vi "Format Alarm Data.vi"(5 "Area color settings":T3(array[cluster]), 7 "Alarm Display Format":T2(array[ring])=[enum."alarm URL"], 8 "Error In":errorcluster, 10 "alarm instances":T1(array[cluster]), 11 "Multicolumn Listbox":refnum<vi>) -> (0 "Error Out":errorcluster, 1 "Alarm Summary Data":string[][](array[string]), 2 "Alarm Summary Headers":string[](array[string]), 3 "dup Multicolumn Listbox":refnum<vi>)   [LabVIEW 2018, in "Dynamic Shared Variables.lvlib"]
doc: "This VI formats alarm data and inserts it into a multicolumn list box."
uses:
  Dynamic Shared Variables.lvlib
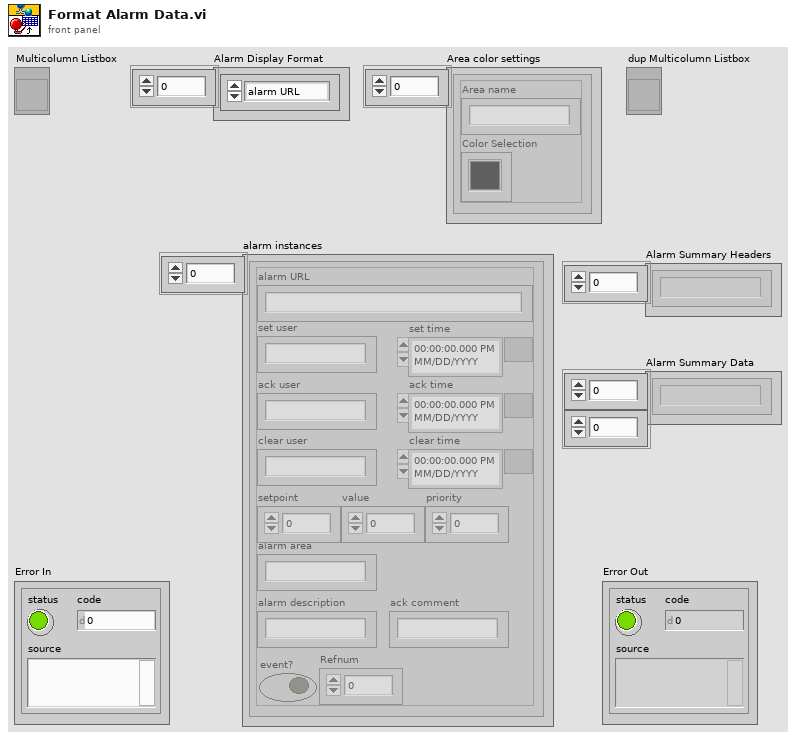
[diagram p1: front panel]
types:
  T1 = cluster{"alarm URL":string, "set time":timestamp, "set user":string, "ack time":timestamp, "ack user":string, "clear time":timestamp, "clear user":string, "setpoint":dbl, "value":dbl, "priority":u32, "alarm area":string, "alarm description":string, "ack comment":string, "event?":bool, "Refnum":u64}[]
  T2 = enum16{"alarm URL", "event?", "set time", "ack time", "clear time", "set user", "ack user", "clear user", "set point", "value", "priority", "alarm area", "alarm description", "ack comment"}[]
  T3 = cluster{"Area name":string, "Color Selection":u32}[]
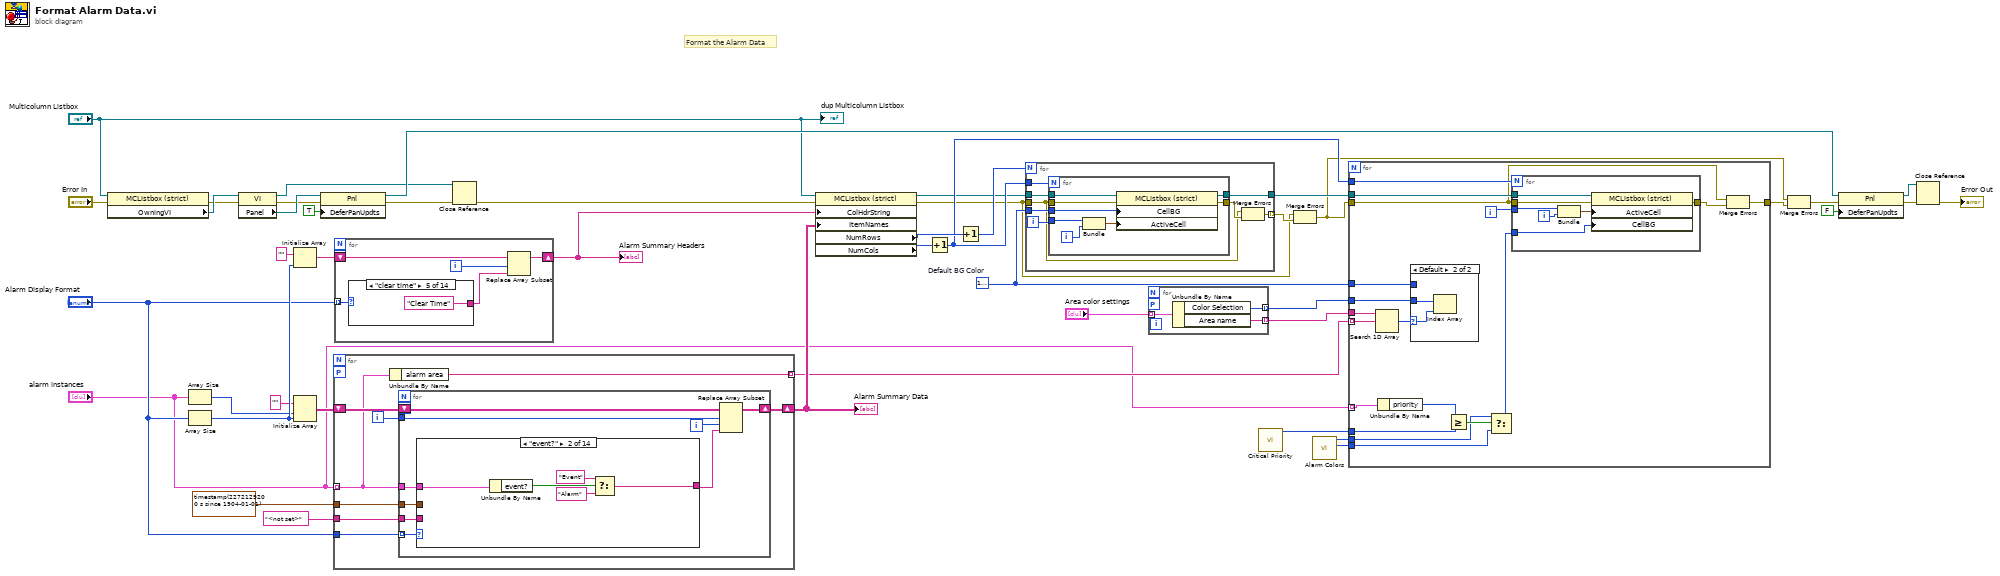
[diagram p0: block diagram]
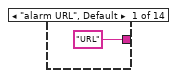
[diagram p3: hidden frame]
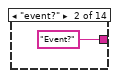
[diagram p4: hidden frame]
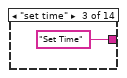
[diagram p5: hidden frame]
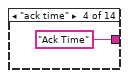
[diagram p6: hidden frame]
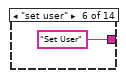
[diagram p7: hidden frame]
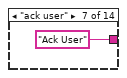
[diagram p8: hidden frame]
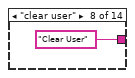
[diagram p9: hidden frame]
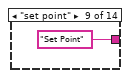
[diagram p10: hidden frame]
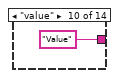
[diagram p11: hidden frame]
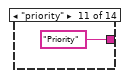
[diagram p12: hidden frame]
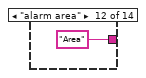
[diagram p13: hidden frame]
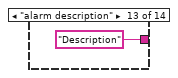
[diagram p14: hidden frame]
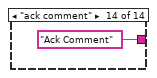
[diagram p15: hidden frame]
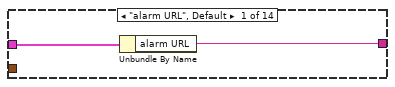
[diagram p16: hidden frame]
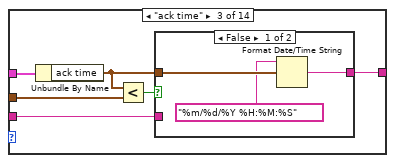
[diagram p17: hidden frame]
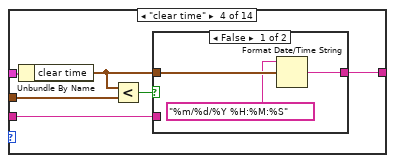
[diagram p19: hidden frame]
diagram:
  w13 = u32 16777226  # Default BG Color
  # "Format the Alarm Data"
  n1 = property class="MCListbox (strict)"(reference="Multicolumn Listbox", error in="Error In") -> (error out=w25:errorcluster, "OwningVI"=w26:refnum<vi>)  [unwired: 1 out]
  n2 = Array Size(array="alarm instances") -> (size(s)=w38:i32)
  n3 = Array Size(array="Alarm Display Format") -> (size(s)=w43:i32)
  n4 = property class="VI"(reference=w26, error in=w25) -> (reference out=w19:refnum<vi>, error out=w23:errorcluster, "Panel"=w24:refnum<vi>)
  n5 = Initialize Array("" ("element"), w43) -> (w44:string[])
  n6 = Initialize Array("" ("alarm URL"), w38, w43) -> (w40:string[][])
  n7 = property class="Pnl"(reference=w24, error in=w23, "DeferPanUpdts"=TRUE ("Defer Panel Updates")) -> (reference out=w20:refnum<vi>, error out=w18:errorcluster)
  n8 = for {
    tunnel: "alarm instances" -> [w48] mode=indexing
    tunnel: "Alarm Display Format" -> [w54]
    shift-right: [w52] -> w45
    shift-left: w40 -> [w53]
    tunnel: timestamp(2272129200 s since 1904-01-01) ("ack time") -> [w50]
    tunnel: "<not set>" ("date/time string") -> [w49]
    tunnel: [w47] -> w35 mode=indexing
    workers-P: _ -> [_]
    i -> [w51]
    n9 = Unbundle By Name(w48) -> ("alarm area"=w47:string)
    n10 = for {
      tunnel: w54 -> [w63] mode=indexing
      tunnel: w48 -> [w55]
      tunnel: w51 -> [w60]
      shift-right: [w61] -> w52
      shift-left: w53 -> [w62]
      tunnel: w50 -> [w57]
      tunnel: w49 -> [w56]
      workers-P: _ -> [_]
      i -> [w59]
      n11 = case shown="\"event?\"" w63 {
        tunnel: w55 -> [w65 w70 w76 w86 w96 w102 w104 w106 w109 w112 w115 w117 w119 w121]
        tunnel: [w64 w66 w75 w85 w95 w101 w103 w105 w107 w110 w113 w116 w118 w120] -> w58
        tunnel: w57 -> [_ _ w73 w83 w93 _ _ _ _ _ _ _ _ _]
        tunnel: w56 -> [_ _ w71 w81 w91 _ _ _ _ _ _ _ _ _]
        frame "alarm URL", Default {
          n12 = Unbundle By Name(w65) -> ("alarm URL"=w64:string)
        }
        frame "event?" {
          n13 = Unbundle By Name(w70) -> ("event?"=w69:bool)
          n14 = Select(t="Event" ("alarm URL"), s=w69, f="Alarm") -> (s? t:f=w66:string)
        }
        frame "ack time" {
          n15 = Unbundle By Name(w76) -> ("ack time"=w72:timestamp)
          n16 = Less?(x=w72, y=w73) -> (x < y?=w74:bool)
          n17 = case shown="False" w74 {
            tunnel: w72 -> [w79 _]
            tunnel: [w77 w80] -> w75
            tunnel: w71 -> [_ w80]
            frame False {
              n18 = Format Date/Time String(time format string (%c)="%m/%d/%Y %H:%M:%S", seconds (now)=w79) -> (date/time string=w77:string)  [unwired: 1 in]
            }
            frame True {
            }
          }
        }
        frame "clear time" {
          n19 = Unbundle By Name(w86) -> ("clear time"=w82:timestamp)
          n20 = Less?(x=w82, y=w83) -> (x < y?=w84:bool)
          n21 = case shown="False" w84 {
            tunnel: w82 -> [w89 _]
            tunnel: [w87 w90] -> w85
            tunnel: w81 -> [_ w90]
            frame False {
              n22 = Format Date/Time String(time format string (%c)="%m/%d/%Y %H:%M:%S", seconds (now)=w89) -> (date/time string=w87:string)  [unwired: 1 in]
            }
            frame True {
            }
          }
        }
        frame "set time" {
          n23 = Unbundle By Name(w96) -> ("set time"=w92:timestamp)
          n24 = Less?(x=w92, y=w93) -> (x < y?=w94:bool)
          n25 = case shown="False" w94 {
            tunnel: w92 -> [w99 _]
            tunnel: [w97 w100] -> w95
            tunnel: w91 -> [_ w100]
            frame False {
              n26 = Format Date/Time String(time format string (%c)="%m/%d/%Y %H:%M:%S", seconds (now)=w99) -> (date/time string=w97:string)  [unwired: 1 in]
            }
            frame True {
            }
          }
        }
        frame "set user" {
          n27 = Unbundle By Name(w102) -> ("set user"=w101:string)
        }
        frame "ack user" {
          n28 = Unbundle By Name(w104) -> ("ack user"=w103:string)
        }
        frame "clear user" {
          n29 = Unbundle By Name(w106) -> ("ack user"=w105:string)
        }
        frame "set point" {
          n30 = Unbundle By Name(w109) -> ("setpoint"=w108:dbl)
          n31 = Number To Fractional String(number=w108) -> (F-format string=w107:string)  [unwired: 3 in]
        }
        frame "value" {
          n32 = Unbundle By Name(w112) -> ("value"=w111:dbl)
          n33 = Number To Fractional String(number=w111) -> (F-format string=w110:string)  [unwired: 3 in]
        }
        frame "priority" {
          n34 = Unbundle By Name(w115) -> ("priority"=w114:u32)
          n35 = Number To Decimal String(number=w114) -> (decimal integer string=w113:string)  [unwired: 1 in]
        }
        frame "alarm area" {
          n36 = Unbundle By Name(w117) -> ("alarm area"=w116:string)
        }
        frame "alarm description" {
          n37 = Unbundle By Name(w119) -> ("alarm description"=w118:string)
        }
        frame "ack comment" {
          n38 = Unbundle By Name(w121) -> ("ack comment"=w120:string)
        }
      }
      n39 = Replace Array Subset(array=w62, new element=w58, index (row)=w60, index (col)=w59) -> (w61:string[][])
    }
  }
  "Alarm Summary Data" <- w45
  n40 = for {
    tunnel: "Alarm Display Format" -> [w126] mode=indexing
    shift-right: [w124] -> w46
    shift-left: w44 -> [w125]
    workers-P: _ -> [_]
    i -> [w123]
    n41 = case shown="\"clear time\"" w126 {
      tunnel: ["URL" ("element") "Event?" ("element") "Set Time" ("element") "Ack Time" ("element") "Clear Time" ("element") "Set User" ("element") "Ack User" ("element") "Clear User" ("element") "Set Point" ("element") "Value" ("element") "Priority" ("element") "Area" ("element") "Description" ("element") "Ack Comment" ("element")] -> w122
      frame "alarm URL", Default {
      }
      frame "event?" {
      }
      frame "set time" {
      }
      frame "ack time" {
      }
      frame "clear time" {
      }
      frame "set user" {
      }
      frame "ack user" {
      }
      frame "clear user" {
      }
      frame "set point" {
      }
      frame "value" {
      }
      frame "priority" {
      }
      frame "alarm area" {
      }
      frame "alarm description" {
      }
      frame "ack comment" {
      }
    }
    n42 = Replace Array Subset(array=w125, new element=w122, index=w123) -> (w124:string[])
  }
  "Alarm Summary Headers" <- w46
  n43 = Close Reference(reference=w19, error in (no error)=w18) -> (error out=w17:errorcluster)
  n44 = property class="MCListbox (strict)"(reference="Multicolumn Listbox", error in=w17, "ColHdrString"=w46, "ItemNames"=w45) -> (reference out=w27:refnum<vi>, error out=w3:errorcluster, "NumRows"=w30:u32, "NumCols"=w31:u32)
  n45 = Increment(x=w31) -> (x+1=w28:u32)
  n46 = Increment(x=w30) -> (x+1=w29:u32)
  n47 = for {
    N: w29 -> [_]
    tunnel: w28 -> [w147]
    tunnel: w27 -> [w146]
    tunnel: w13 -> [w145]
    tunnel: w3 -> [w141]
    tunnel: [w144] -> w14
    tunnel: [w143] -> w4 mode=indexing
    i -> [w148]
    n48 = for {
      N: w147 -> [_]
      tunnel: w148 -> [w156]
      tunnel: [w155] -> w142
      tunnel: w146 -> [w153]
      tunnel: w145 -> [w152]
      tunnel: w141 -> [w151]
      tunnel: [w150] -> w144
      i -> [w154]
      n49 = Bundle(w156, w154) -> (w149:cluster{i32, i32})  [unwired: 1 in]
      n50 = property class="MCListbox (strict)"(reference=w153, error in=w151, "CellBG"=w152, "ActiveCell"=w149) -> (reference out=w150:refnum<vi>, error out=w155:errorcluster)
    }
    n51 = Merge Errors(w141, w142) -> (w143:errorcluster)
  }
  n52 = for {
    tunnel: "Area color settings" -> [w159] mode=indexing
    tunnel: [w158] -> w33 mode=indexing
    tunnel: [w157] -> w32 mode=indexing
    workers-P: _ -> [_]
    n53 = Unbundle By Name(w159) -> ("Color Selection"=w157:u32, "Area name"=w158:string)
  }
  n54 = call "Critical Priority.vi"() -> ("critical priority"=w8:i32)  [unwired: 11 in]
  n55 = Merge Errors(w3, w4) -> (w1:errorcluster)
  n56 = call "Alarm Colors.vi"() -> ("Non-critical"=w6:u32, "Critical"=w7:u32)  [unwired: 10 in]
  n57 = for {
    tunnel: w14 -> [w177]
    tunnel: w35 -> [w174] mode=indexing
    tunnel: [w162] -> w2
    tunnel: w28 -> [w176]
    tunnel: w33 -> [w175]
    tunnel: w32 -> [w173]
    tunnel: w1 -> [w160]
    tunnel: w13 -> [w171]
    tunnel: "alarm instances" -> [w169] mode=indexing
    tunnel: w8 -> [w167]
    tunnel: w7 -> [w165]
    tunnel: w6 -> [w164]
    i -> [w170]
    n58 = Search 1D Array(1D array=w175, element=w174) -> (index of element=w172:i32)  [unwired: 1 in]
    n59 = Unbundle By Name(w169) -> ("priority"=w168:u32)
    n60 = case shown="Default" w172 {
      selector: w172 -> [_ w178]
      tunnel: w173 -> [_ w179]
      tunnel: w171 -> [_ _]
      frame ..-1 {
      }
      frame Default {
        n61 = Index Array(array=w179, index=w178) -> ()  [unwired: 1 out]
      }
    }
    n62 = Greater Or Equal?(x=w168, y=w167) -> (x >= y?=w166:bool)
    n63 = Select(t=w165, s=w166, f=w164) -> (s? t:f=w163:u32)
    n64 = for {
      N: w176 -> [_]
      tunnel: w177 -> [w186]
      tunnel: w170 -> [w185]
      tunnel: [w184] -> w161
      tunnel: w163 -> [w181]
      tunnel: w160 -> [w180]
      i -> [w183]
      n65 = Bundle(w185, w183) -> (w182:cluster{i32, i32})  [unwired: 1 in]
      n66 = property class="MCListbox (strict)"(reference=w186, error in=w180, "ActiveCell"=w182, "CellBG"=w181) -> (error out=w184:errorcluster)  [unwired: 1 out]
    }
    n67 = Merge Errors(w160, w161) -> (w162:errorcluster)
  }
  n68 = Merge Errors(w1, w2) -> (w5:errorcluster)
  n69 = property class="Pnl"(reference=w20, error in=w5, "DeferPanUpdts"=FALSE ("Defer Panel Updates")) -> (reference out=w15:refnum<vi>, error out=w16:errorcluster)
  n70 = Close Reference(reference=w15, error in (no error)=w16) -> (error out=→"Error Out":errorcluster)
  "dup Multicolumn Listbox" <- "Multicolumn Listbox"
